vi "query_components.vi"(8 "error in (no error)":errorcluster, 9 "part":string, 11 "DB Session ID":i32) -> (0 "error out":errorcluster, 1 "Components":T1[](array[typedef]), 3 "DB Session ID out":i32)   [LabVIEW 2017, in "Database.lvlib"]
uses:
  Database.lvlib
  DB Component.ctl
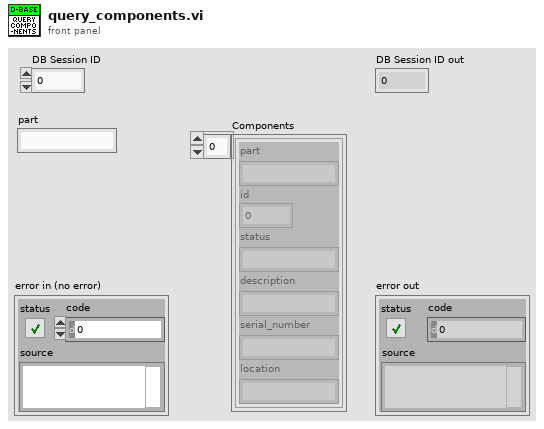
[diagram p1: front panel]
types:
  T1 = typedef "Database.lvlib/DB Component.ctl" = cluster{"part":string, "id":i32, "status":string, "description":string, "serial_number":string, "location":string}
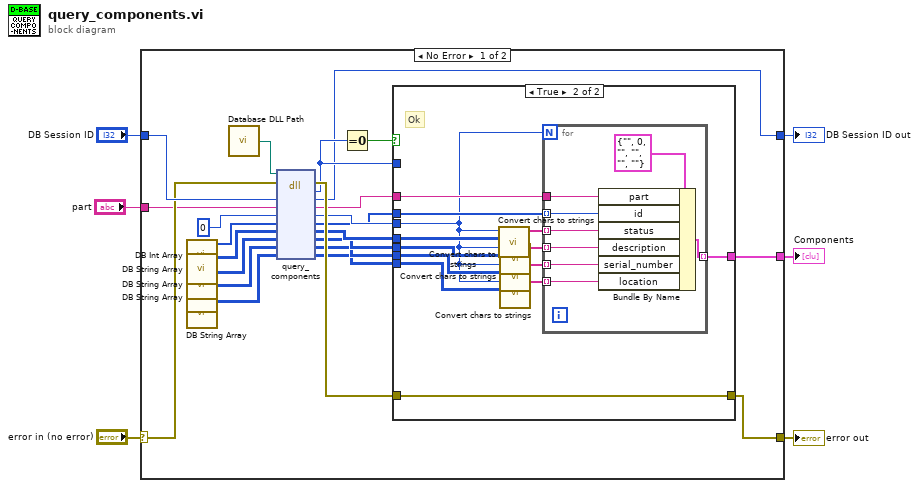
[diagram p0: block diagram]
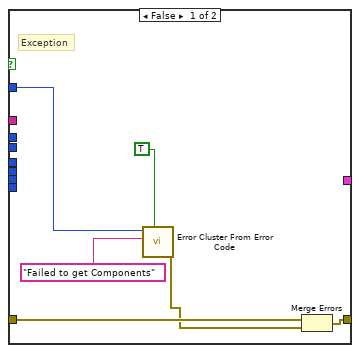
[diagram p2: hidden frame]
diagram:
  n1 = case shown="No Error" "error in (no error)" {
    selector: "error in (no error)" -> [w26 w58]
    tunnel: [w25 w58] -> w4
    tunnel: "DB Session ID" -> [w27 w57]
    tunnel: [w22 _] -> w1
    tunnel: [w20 w57] -> w3
    tunnel: "part" -> [w15 _]
    frame No Error {
      n2 = call "DB Int Array.vi"() -> ("DB Int Array"=w13:i32[])  [unwired: 11 in]
      n3 = call "DB String Array.vi"() -> ("DB string array"=w12:i8[][])  [unwired: 11 in]
      n4 = call "DB String Array.vi"() -> ("DB string array"=w11:i8[][])  [unwired: 11 in]
      n5 = call "DB String Array.vi"() -> ("DB string array"=w10:i8[][])  [unwired: 11 in]
      n6 = call "DB String Array.vi"() -> ("DB string array"=w9:i8[][])  [unwired: 11 in]
      n7 = call "Database DLL Path.vi"() -> ("DLL Path"=w28:path)  [unwired: 5 in]
      n8 = dll-call lib="?" fn="query_components"(path in=w28, error in=w26, "session_id"=w27, "part"=w15, "n_component"=0, "id"=w13, "status"=w12, "description"=w11, "serial_number"=w10, "location"=w9) -> (error out=w29:errorcluster, "return type"=w21:i32, "session_id"=w20:i32, "part"=w23:string, "n_component"=w19:i32, "id"=w8:i32[], "status"=w18:i8[][], "description"=w17:i8[][], "serial_number"=w16:i8[][], "location"=w7:i8[][])  [unwired: 1 in, 1 out]
      n9 = Equal To 0?(x=w21) -> (x = 0?=w24:bool)
      n10 = case shown="True" w24 {
        tunnel: w29 -> [w35 w48]
        tunnel: [w34 w48] -> w25
        tunnel: w23 -> [_ w40]
        tunnel: [_ w47] -> w22
        tunnel: w21 -> [w30 _]
        tunnel: w19 -> [_ w36]
        tunnel: w18 -> [_ w46]
        tunnel: w17 -> [_ w44]
        tunnel: w16 -> [_ w42]
        tunnel: w8 -> [_ w39]
        tunnel: w7 -> [_ w37]
        frame False {
          # "Exception"
          n11 = call <vilib>:"Error Cluster From Error Code.vi"("show call chain? (False)"=TRUE, "error message (\"\")"="Failed to get Components" ("error message (\"\")"), "error code (0)"=w30) -> ("error out"=w33:errorcluster)  [unwired: 6 in]
          n12 = Merge Errors(w35, w33) -> (w34:errorcluster)
        }
        frame True {
          # "Ok"
          n13 = call "Convert chars to strings.vi"("Char Array"=w46, "Array Length"=w36) -> ("Strings"=w45:string[])  [unwired: 9 in]
          n14 = call "Convert chars to strings.vi"("Char Array"=w44, "Array Length"=w36) -> ("Strings"=w43:string[])  [unwired: 9 in]
          n15 = call "Convert chars to strings.vi"("Char Array"=w42, "Array Length"=w36) -> ("Strings"=w41:string[])  [unwired: 9 in]
          n16 = call "Convert chars to strings.vi"("Char Array"=w37, "Array Length"=w36) -> ("Strings"=w38:string[])  [unwired: 9 in]
          n17 = for {
            N: w36 -> [_]
            tunnel: [w56] -> w47 mode=indexing
            tunnel: w45 -> [w52] mode=indexing
            tunnel: w43 -> [w51] mode=indexing
            tunnel: w41 -> [w50] mode=indexing
            tunnel: w40 -> [w54]
            tunnel: w39 -> [w53] mode=indexing
            tunnel: w38 -> [w49] mode=indexing
            n18 = Bundle By Name(cluster=T1 {"part"="", "id"=0, "status"="", "description"="", "serial_number"="", "location"=""} ("Cluster"), "part"=w54, "id"=w53, "status"=w52, "description"=w51, "serial_number"=w50, "location"=w49) -> (w56:T1)
          }
        }
      }
    }
    frame Error {
    }
  }
  "error out" <- w4
  "DB Session ID out" <- w3
  "Components" <- w1
